vi "Notify Fatal Error.vi"(8 "error in (no error)":errorcluster, 10 "error":string, 11 "Master Controller in":refnum<class "Master Controller.lvclass">) -> (0 "error out":errorcluster, 3 "Master Controller out":refnum<class "Master Controller.lvclass">)   [LabVIEW 2015, in "Master Controller Core.lvlib" / "Master Controller.lvclass"]
uses:
  Master Controller.lvclass
  Communications/SCADA Communcations Actor/SCADA Communications/Controls/EMS Message Cluster.ctl
  Master Controller.lvclass/Master Controller.ctl
  Communications/SCADA Communcations Actor/SCADA Communications Messages/Transmit EMS Message Msg/Transmit EMS Message Msg.lvclass/Transmit EMS Message Msg.ctl
  <vilib>/ActorFramework/Message Enqueuer/Message Enqueuer.lvclass/Message Enqueuer.ctl
  <vilib>/ActorFramework/Actor/Actor.lvclass/Actor.ctl
  <vilib>/ActorFramework/Message Enqueuer/Enqueue.vi
  <vilib>/ActorFramework/Message Enqueuer/Init from Existing Queue.vi
  <vilib>/ActorFramework/Message Priority Queue/Priority Enqueue.vi
  Communications/SCADA Communcations Actor/SCADA Communications Messages/Transmit EMS Message Msg/Transmit EMS Message Msg.lvclass
  <vilib>/ActorFramework/Message Enqueuer/Message Enqueuer.lvclass
  <vilib>/ActorFramework/Stop Msg/Stop Msg.lvclass
  Communications/SCADA Communcations Actor/SCADA Communications/SCADA Communications.lvclass
  Utilities/Message Strings.llb/Message String Utilities.lvlib
  <vilib>/ActorFramework/Actor/Actor.lvclass
  Utilities/Status Messaging.llb/Status Messaging.lvlib
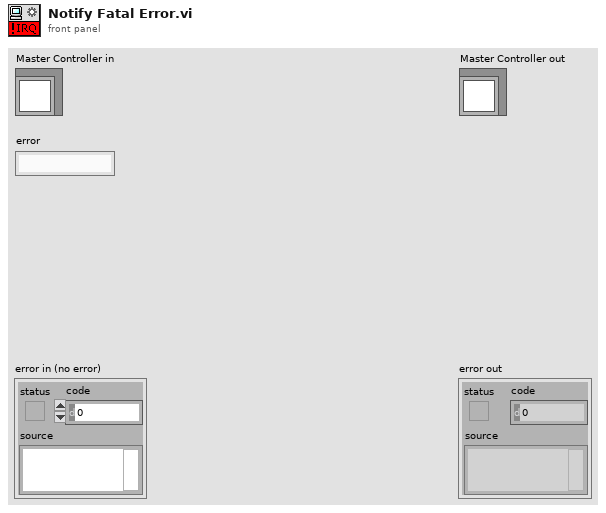
[diagram p1: front panel]
types:
  T1 = typedef "SCADA Communcations Actor.lvlib/SCADA Communications.lvclass/EMS Message Cluster.ctl" = cluster{"Name":string, "Content":string}
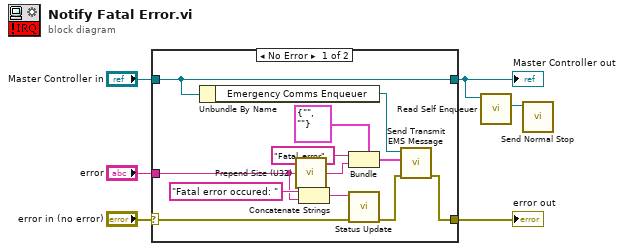
[diagram p0: block diagram]
diagram:
  n1 = case shown="No Error" "error in (no error)" {
    selector: "error in (no error)" -> [w11 w20]
    tunnel: [w13 w20] -> w4
    tunnel: [w14 w19] -> w2
    tunnel: "Master Controller in" -> [w14 w19]
    tunnel: "error" -> [w8 _]
    frame No Error {
      n2 = Unbundle By Name(w14) -> ("Emergency Comms Enqueuer"=w16:refnum<class "Message Enqueuer.lvclass">)
      n3 = call "Prepend Size (U32).vi"("String in"=w8) -> ("String out"=w12:string)
      n4 = Concatenate Strings("Fatal error occured: " ("Name"), w8) -> (w7:string)
      n5 = Bundle(cluster=T1 {"Name"="", "Content"=""} ("Message"), "Name"="Fatal_error", "Content"=w12) -> (w17:T1)
      n6 = call "Status Update.vi"("error in (no error)"=w11, "Status Update"=w7) -> ("error out"=w10:errorcluster)  [unwired: 8 in, 1 out]
      n7 = call "Send Transmit EMS Message.vi"("error in (no error)"=w10, "Message"=w17, "Message Enqueuer"=w16) -> ("error out"=w13:errorcluster)  [unwired: 7 in, 1 out]
    }
    frame Error {
    }
  }
  "error out" <- w4
  "Master Controller out" <- w2
  n8 = call <vilib>:"Read Self Enqueuer.vi"("Actor"=w2) -> ("Self Enqueuer"=w1:refnum<class "Message Enqueuer.lvclass">)  [unwired: 10 in]
  n9 = call <vilib>:"Send Normal Stop.vi"("Message Enqueuer"=w1) -> ()  [unwired: 10 in, 1 out]
